vi "Save Library Documentation.vi"(9 "New Description":string, 10 "DQMH Modules Info In":T1, 11 "Library in":refnum<vi>) -> (0 "error out":errorcluster, 2 "DQMH Modules Info Out":T1, 3 "Lib out":refnum<vi>)   [LabVIEW 2019, in "Panther Dashboard.lvlib"]
uses:
  Panther Dashboard.lvlib
  DQMH Modules Info--cluster.ctl
  Module type--enum.ctl
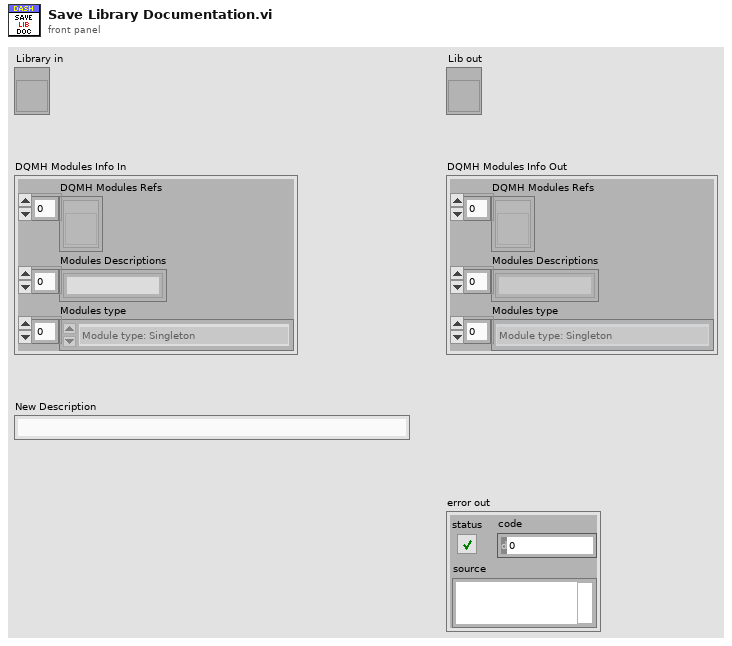
[diagram p1: front panel]
types:
  T1 = typedef "Panther Dashboard.lvlib/DQMH Modules Info--cluster.ctl" = cluster{"DQMH Modules Refs":refnum<vi>[], "Modules Descriptions":string[], "Modules type":T2[]}
  T2 = typedef "Panther Dashboard.lvlib/Module type--enum.ctl" = enum16{"Module type: Singleton", "Module type: Cloneable"}
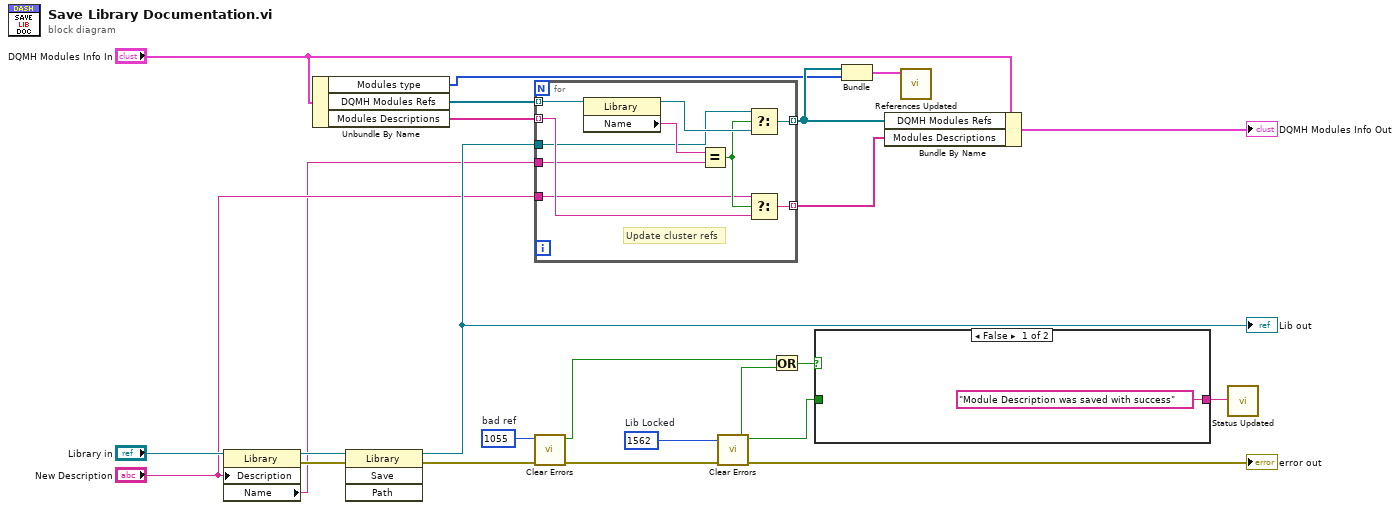
[diagram p0: block diagram]
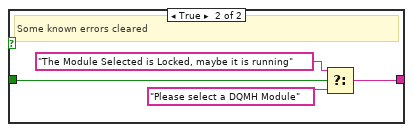
[diagram p2: hidden frame]
diagram:
  w5 = 1562  # Lib Locked
  w6 = 1055  # bad ref
  n1 = property class="Library"(reference="Library in", "Description"="New Description") -> (reference out=w16:refnum<vi>, error out=w23:errorcluster, "Name"=w8:string)  [unwired: 1 in]
  n2 = Unbundle By Name("DQMH Modules Info In") -> ("Modules type"=w2:T2[], "DQMH Modules Refs"=w17:refnum<vi>[], "Modules Descriptions"=w11:string[])
  n3 = invoke class="Library" method="Save"(reference=w16, error in=w23) -> (reference out=w12:refnum<vi>, error out=w22:errorcluster)  [unwired: 2 in, 2 out]
  "Lib out" <- w12
  n4 = for {
    tunnel: w17 -> [w33] mode=indexing
    tunnel: [w30] -> w14 mode=indexing
    tunnel: w12 -> [w24]
    tunnel: w11 -> [w28] mode=indexing
    tunnel: [w27] -> w10 mode=indexing
    tunnel: "New Description" -> [w26]
    tunnel: w8 -> [w25]
    # "Update cluster refs"
    n5 = property class="Library"(reference=w33) -> (reference out=w31:refnum<vi>, "Name"=w32:string)  [unwired: 1 in, 1 out]
    n6 = Equal?(x=w32, y=w25) -> (x = y?=w29:bool)
    n7 = Select(t=w24, s=w29, f=w31) -> (s? t:f=w30:refnum<vi>)
    n8 = Select(t=w26, s=w29, f=w28) -> (s? t:f=w27:string)
  }
  n9 = call <vilib>:"Clear Errors.vi"("error in (no error)"=w22, "specific error code to clear (0: all)"=w6) -> ("error out"=w21:errorcluster, "specific error cleared?"=w7:bool)  [unwired: 4 in]
  n10 = call <vilib>:"Clear Errors.vi"("error in (no error)"=w21, "specific error code to clear (0: all)"=w5) -> ("error out"=→"error out":errorcluster, "specific error cleared?"=w3:bool)  [unwired: 4 in]
  n11 = Or(x=w7, y=w3) -> (x .or. y?=w4:bool)
  n12 = case shown="False" w4 {
    tunnel: w3 -> [_ w38]
    tunnel: ["Module Description was saved with success" ("Status") w35] -> w1
    frame False {
    }
    frame True {
      # "Some known errors cleared"
      n13 = Select(t="The Module Selected is Locked, maybe it is running" ("Status"), s=w38, f="Please select a DQMH Module" ("Status")) -> (s? t:f=w35:string)
    }
  }
  n14 = Bundle(w14, "Modules type"=w2) -> (w18:cluster{refnum<vi>[], "Modules type":T2[]})  [unwired: 1 in]
  n15 = Bundle By Name(cluster="DQMH Modules Info In", "DQMH Modules Refs"=w14, "Modules Descriptions"=w10) -> (→"DQMH Modules Info Out":T1)
  n16 = call "References Updated.vi"("DQMH Refs"=w18) -> ()  [unwired: 10 in, 1 out]
  n17 = call "Status Updated.vi"("Status"=w1) -> ()  [unwired: 10 in, 1 out]
